vi "uActor_Exec.vi"(6 "Original uMsg":refnum<class "uMsg.lvclass">, 8 "error in (no error)":errorcluster, 9 "Data":refnum<class "uData.lvclass">, 10 "Command":string, 11 "uView in":refnum<class "uView.lvclass">) -> (0 "error out":errorcluster, 1 "reply":refnum<class "uData.lvclass">, 3 "uView out":refnum<class "uView.lvclass">)   [LabVIEW 2023, in "uLib.lvlib" / "uView.lvclass"]
doc: "uObserver actor by default ignores any output wired to the output terminal 'reply' in the child override EXEC method unless the child class invokes the uActor_EnableAutoAck method."
uses:
  uView.lvclass
  uData/uData/uData.lvclass
  uMsg/uMsg/uMsg.lvclass
  uView.lvclass/uView.ctl
  uData/uData/uData.lvclass/uData.ctl
  uData/uData/Condition Tag Name.vi
  uData/uData/Blank Key Reserved String.vi
  uObserver/uObserver.lvclass
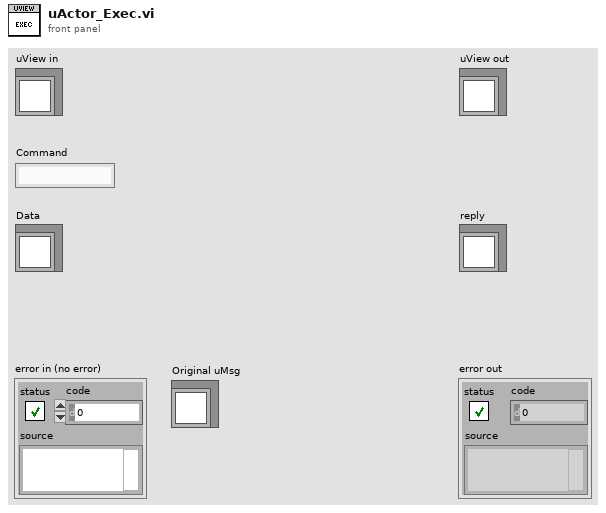
[diagram p1: front panel]
types:
  T1 = enum32{"Invalid", "Standard", "Closed", "Hidden", "Minimized", "Maximized"}
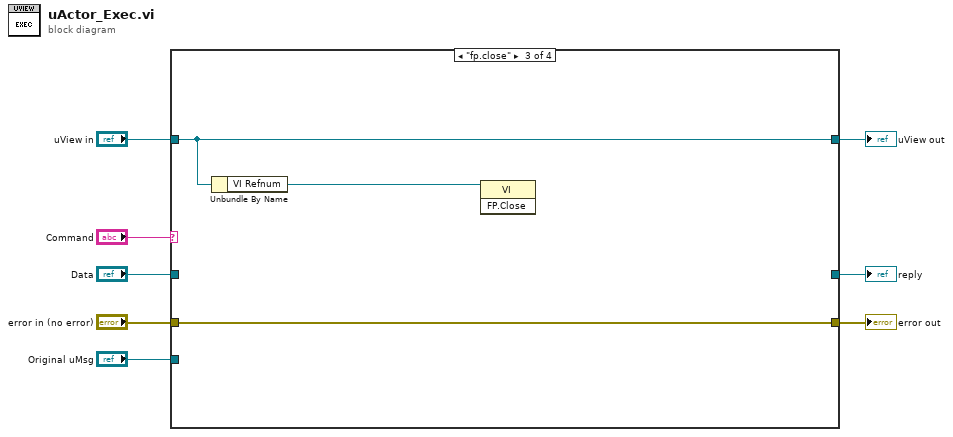
[diagram p0: block diagram]
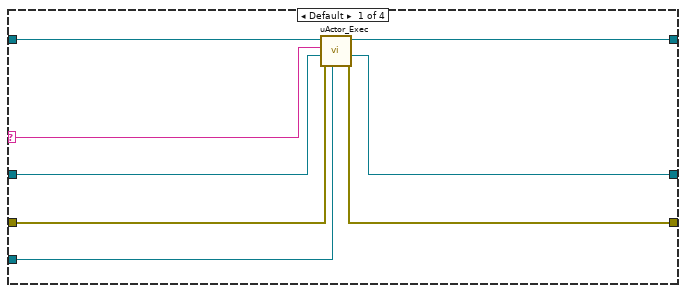
[diagram p2: hidden frame]
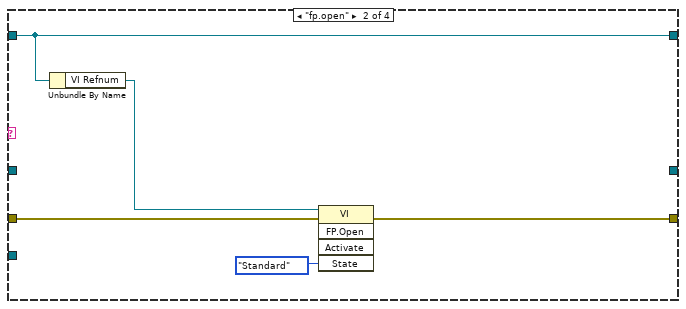
[diagram p3: hidden frame]
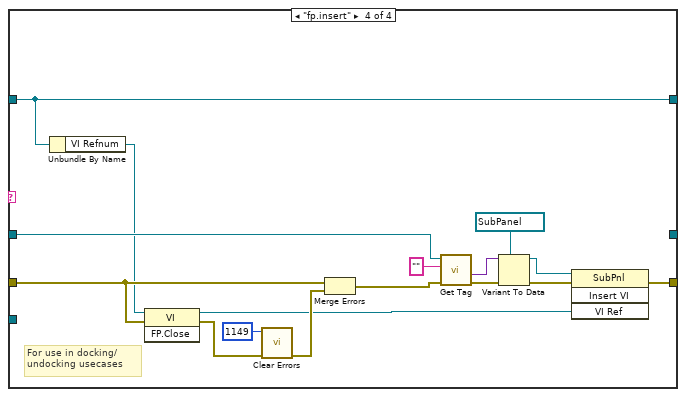
[diagram p4: hidden frame]
diagram:
  n1 = case shown="\"fp.close\"" "Command" {
    selector: "Command" -> [w9 _ _ _]
    tunnel: [w16 w19 w22 w36] -> w8
    tunnel: [w15 _ _ _] -> w7
    tunnel: [w14 w21 w24 w37] -> w6
    tunnel: "Original uMsg" -> [w13 _ _ _]
    tunnel: "error in (no error)" -> [w12 w18 w22 w40]
    tunnel: "Data" -> [w11 _ _ w31]
    tunnel: "uView in" -> [w10 w21 w24 w37]
    frame Default {
      n2 = call-parent "uActor_Exec.vi"("Original uMsg"=w13, "error in (no error)"=w12, "Data"=w11, "Command"=w9, "uObserver in"=w10) -> ("error out"=w16:errorcluster, "reply"=w15:refnum<class "uData.lvclass">, "uObserver out"=w14:refnum<class "uView.lvclass">)  [unwired: 4 in]
    }
    frame "fp.open" {
      n3 = Unbundle By Name(w21) -> ("VI Refnum"=w20:refnum<vi>)
      n4 = invoke class="VI" method="FP.Open"(reference=w20, error in=w18, "State"=T1."Standard") -> (error out=w19:errorcluster)  [unwired: 2 in, 4 out]
    }
    frame "fp.close" {
      n5 = Unbundle By Name(w24) -> ("VI Refnum"=w23:refnum<vi>)
      n6 = invoke class="VI" method="FP.Close"(reference=w23) -> ()  [unwired: 2 in, 3 out]
    }
    frame "fp.insert" {
      # "For use in docking/undocking usecases"
      n7 = Unbundle By Name(w37) -> ("VI Refnum"=w28:refnum<vi>)
      n8 = invoke class="VI" method="FP.Close"(reference=w28, error in=w40) -> (reference out=w27:refnum<vi>, error out=w26:errorcluster)  [unwired: 1 in, 1 out]
      n9 = call <vilib>:"Clear Errors.vi"("error in (no error)"=w26, "specific error code to clear (0: all)"=1149) -> ("error out"=w39:errorcluster)  [unwired: 4 in, 1 out]
      n10 = Merge Errors(w40, w39) -> (w25:errorcluster)
      n11 = call "Get Tag.vi"("error in (no error)"=w25, "tag (case insensitive)"="", "uData in"=w31) -> ("error out"=w38:errorcluster, "value"=w32:variant)  [unwired: 5 in, 2 out]
      n12 = Variant To Data(error in=w38, type=refnum<vi> refnum ("reference out"), Variant=w32) -> (data=w34:refnum<vi>, error out=w35:errorcluster)
      n13 = invoke class="SubPnl" method="Insert VI"(reference=w34, error in=w35, "VI Ref"=w27) -> (error out=w36:errorcluster)  [unwired: 1 in, 3 out]
    }
  }
  "error out" <- w8
  "uView out" <- w6
  "reply" <- w7
